vi "WaitForUnwind.vi"(8 "Error In":errorcluster, 11 "AutoData":T1) -> (0 "Error Out":errorcluster, 3 "AutoData out":T1)   [LabVIEW 2019, in "AutoMode.lvlib"]
uses:
  AutoMode.lvlib
  Cluster - AutoModeData.ctl
  MainController/Cluster - TestSettings.ctl
  MainController/Cluster - HardwareConfiguration.ctl
  MainController/Cluster - TestResults.ctl
  Cluster - AutoModeMessage.ctl
  Enum - AutoModeState.ctl
  MainController/Cluster - MainControllerMessage.ctl
  MainController/Enum - MainState.ctl
  Mark10 API/ReadTravelAndForce.vi
  Mark10 API/Mark 10 TSTM-DC.lvlib
  MainController/MainController.lvlib
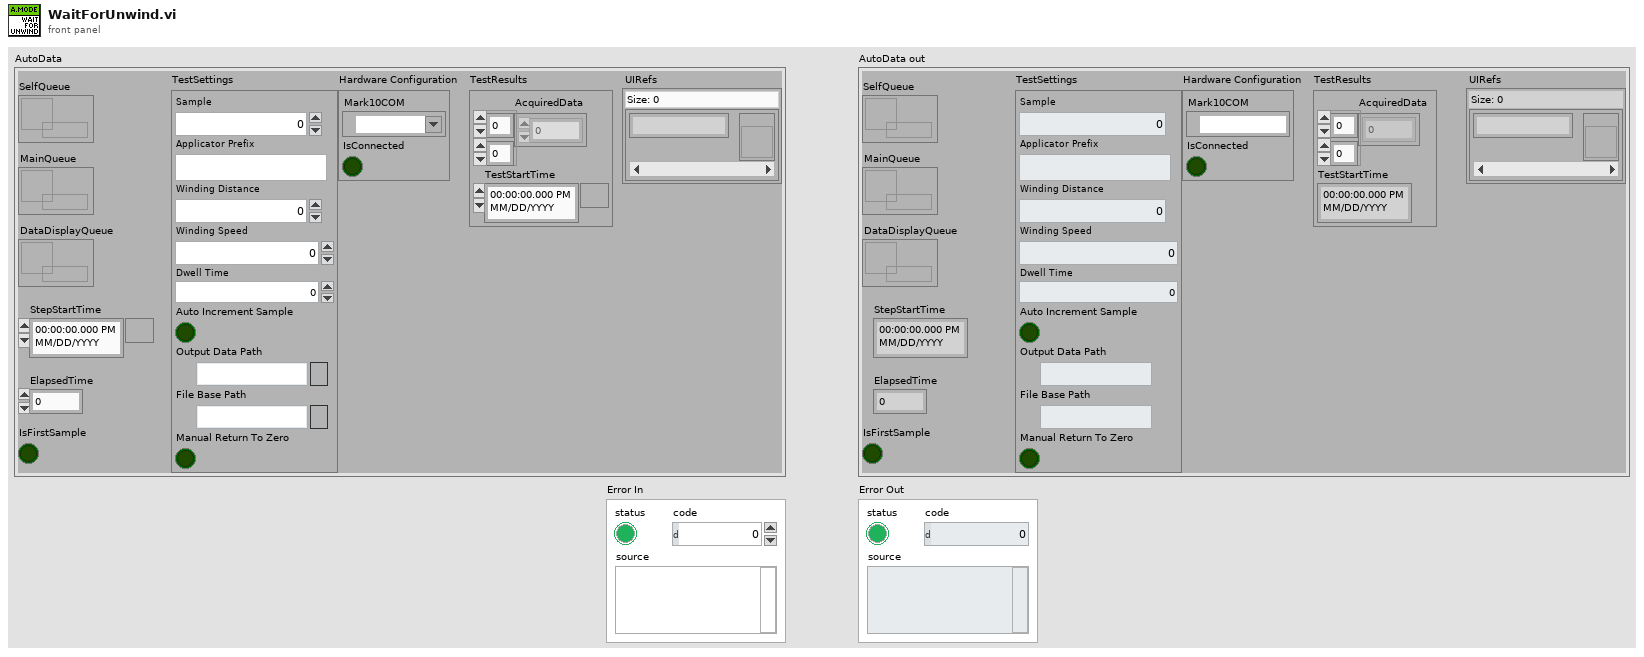
[diagram p1: front panel]
types:
  T1 = typedef "AutoMode.lvlib/Cluster - AutoModeData.ctl" = cluster{"DataDisplayQueue":refnum<queue>, "StepStartTime":timestamp, "TestSettings":T2, "Hardware Configuration":T3, "TestResults":T4, "ElapsedTime":dbl, "IsFirstSample":bool, "SelfQueue":refnum<queue>, "MainQueue":refnum<queue>, "UIRefs":map{string, refnum<vi>}}
  T2 = typedef "MainController.lvlib/Cluster - TestSettings.ctl" = cluster{"Sample":u32, "Applicator Prefix":string, "Winding Distance":dbl, "Winding Speed":dbl, "Dwell Time":dbl, "Auto Increment Sample":bool, "Output Data Path":path, "File Base Path":path, "Manual Return To Zero":bool}
  T3 = typedef "MainController.lvlib/Cluster - HardwareConfiguration.ctl" = cluster{"Mark10COM":refnum<visa-resource-name>, "IsConnected":bool}
  T4 = typedef "MainController.lvlib/Cluster - TestResults.ctl" = cluster{"AcquiredData":dbl[][], "TestStartTime":timestamp}
  T5 = typedef "AutoMode.lvlib/Enum - AutoModeState.ctl" = enum16{"Initialize", "Idle", "UpdateConfig", "UpdateHWConfig", "BroadcastSettings", "Start", "CheckValidReportPath", "Winding", "WaitForWinding", "Unwind", "WaitForUnwind", "Stop", "Abort", "WriteDataToFile", "EventTriggered", "GenerateFilePath", "ZeroPosition", "GotoZero", "Error", "Exit"}
  T6 = typedef "Mark 10 TSTM-DC.lvlib/Cluster - FeedbackData.ctl" = cluster{"Angle":dbl, "Torque":dbl, "Work":dbl}
  T7 = cluster{"number: 0 to 1":dbl, "number: 0 to 1":dbl, "number: 0 to 1":dbl}
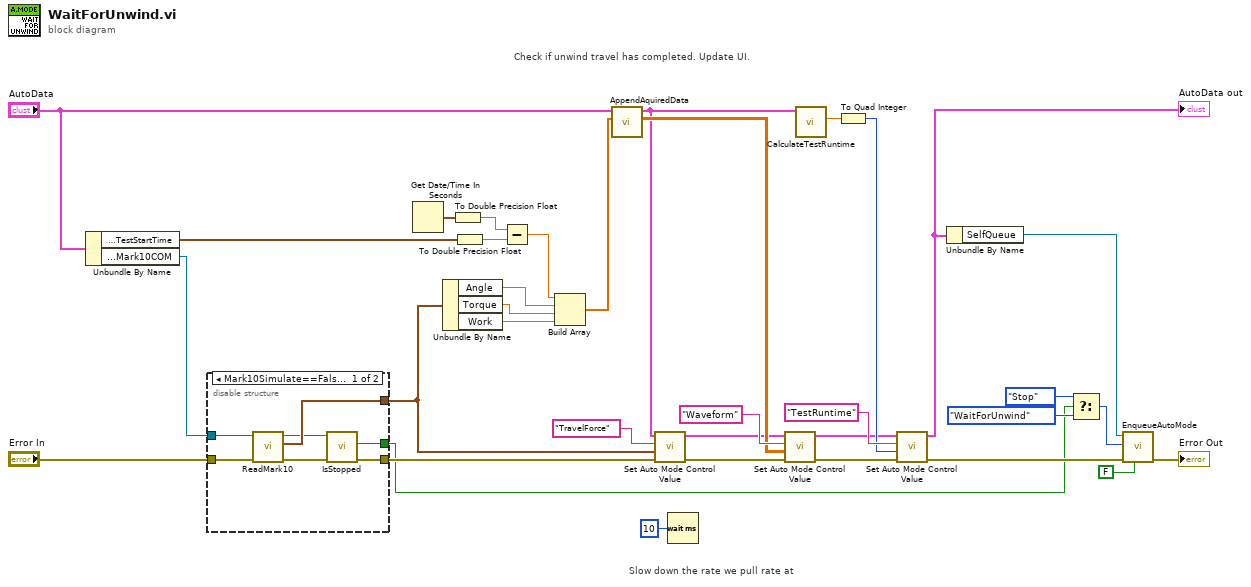
[diagram p0: block diagram]
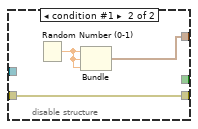
[diagram p2: hidden frame]
diagram:
  # "Check if unwind travel has completed. Update UI."
  # "Slow down the rate we pull rate at"
  n1 = Unbundle By Name("AutoData") -> ("TestResults.TestStartTime"=w7:timestamp, "Hardware Configuration.Mark10COM"=w5:refnum<visa-resource-name>)
  n2 = disable-structure shown="Mark10Simulate==False, Default" {
    disable-tunnel: w5 -> [w42 _]
    disable-tunnel: "Error In" -> [w41 w45]
    disable-tunnel: [w38 w45] -> w4
    disable-tunnel: [w39 w43] -> w3
    disable-tunnel: [w36 _] -> w1
    frame condition #0 (active) {
      n3 = call-poly "ReadMark10.vi"("error in"=w41, "VISA resource name"=w42) -> ("error out"=w40:errorcluster, "FeedbackData"=w39:T6, "VISA resource name out"=w37:refnum<visa-resource-name>)  [unwired: 7 in]
      n4 = call "IsStopped.vi"("Error In"=w40, "VISA resource name"=w37) -> ("Error Out"=w38:errorcluster, "IsStopped"=w36:bool)  [unwired: 7 in, 1 out]
    }
    frame condition #1 {
      n5 = Random Number (0-1)() -> (number: 0 to 1=w44:dbl)
      n6 = Bundle("number: 0 to 1"=w44, "number: 0 to 1"=w44, "number: 0 to 1"=w44) -> (w43:T7)  [unwired: 1 in]
    }
  }
  n7 = Get Date/Time In Seconds() -> (seconds since 1Jan1904=w32:timestamp)
  n8 = Unbundle By Name(w3) -> ("Angle"=w33:dbl, "Torque"=w34:dbl, "Work"=w35:dbl)
  n9 = To Double Precision Float(number=w32) -> (double precision float=w26:dbl)
  n10 = To Double Precision Float(number=w7) -> (double precision float=w25:dbl)
  n11 = Subtract(x=w26, y=w25) -> (x-y=w24:dbl)
  n12 = Build Array(w24, w33, w34, w35) -> (w30:dbl[])
  n13 = call "AppendAquiredData.vi"("Array"=w30, "CycleTestData in"="AutoData") -> ("TestData"=w18:dbl[][], "CycleTestData out"=w13:T1)  [unwired: 7 in, 1 out]
  n14 = call "Set Auto Mode Control Value.vi"("Error In"=w4, "Value"=w3, "key"="TravelForce", "AutoData"=w13) -> ("Error Out"=w15:errorcluster, "AutoData out"=w14:T1)  [unwired: 6 in]
  n15 = Wait (ms)(milliseconds to wait=u32 10) -> ()  [unwired: 1 out]
  n16 = call "Set Auto Mode Control Value.vi"("Error In"=w15, "Value"=w18, "key"="Waveform", "AutoData"=w14) -> ("Error Out"=w17:errorcluster, "AutoData out"=w19:T1)  [unwired: 6 in]
  n17 = call "CalculateTestRuntime.vi"("AutoData"=w13) -> ("ElapsedTime"=w23:dbl)  [unwired: 10 in]
  n18 = To Quad Integer(1:w23) -> (0:w21:i64)
  n19 = call "Set Auto Mode Control Value.vi"("Error In"=w17, "Value"=w21, "key"="TestRuntime", "AutoData"=w19) -> ("Error Out"=w11:errorcluster, "AutoData out"=w10:T1)  [unwired: 6 in]
  "AutoData out" <- w10
  n20 = Unbundle By Name(w10) -> ("SelfQueue"=w9:refnum<queue>)
  n21 = Select(t=Enum_-_AutoModeState."Stop" ("CycleTestState"), s=w1, f=Enum_-_AutoModeState."WaitForUnwind" ("CycleTestState")) -> (s? t:f=w27:T5)
  n22 = call "EnqueueAutoMode.vi"("Priority Message"=FALSE, "error in (no error)"=w11, "AutoState"=w27, "Queue in"=w9) -> ("error out"=→"Error Out":errorcluster)  [unwired: 6 in, 1 out]
